vi "save_bin2.vi"(4 "error in":errorcluster, 5 "xz":T1, 7 "start path":path) -> (0 "error out":errorcluster, 1 "timestamp":timestamp, 3 "file path out":path)   [LabVIEW 2010]
uses:
  lib/Global 2.vi
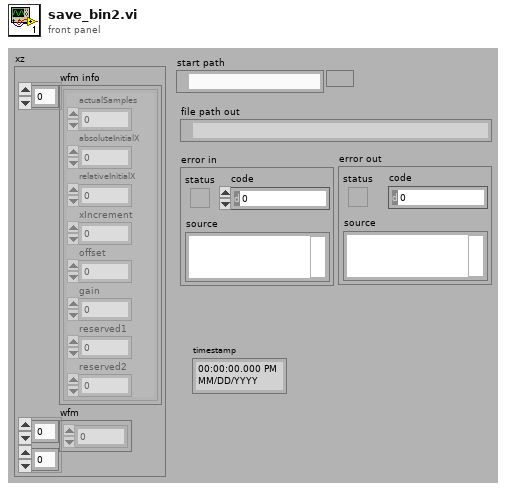
[diagram p1: front panel]
types:
  T1 = cluster{"wfm info":cluster{"actualSamples":i32, "absoluteInitialX":dbl, "relativeInitialX":dbl, "xIncrement":dbl, "offset":dbl, "gain":dbl, "reserved1":dbl, "reserved2":dbl}[], "wfm":i16[][]}
  T2 = enum16{"open", "open or create", "create or replace", "create", "open (read-only)"}
  T3 = cluster{"actualSamples":i32, "absoluteInitialX":dbl, "relativeInitialX":dbl, "xIncrement":dbl, "offset":dbl, "gain":dbl, "reserved1":dbl, "reserved2":dbl}[]
  T4 = cluster{"actualSamples":i32, "absoluteInitialX":dbl, "relativeInitialX":dbl, "xIncrement":dbl, "offset":dbl, "gain":dbl, "reserved1":dbl, "reserved2":dbl}
  T5 = cluster{"name":enum16{"sync", "phase_a", "phase_b", "phase_c", "ground"}, "num":i32, "Numeric":i32}[]
  T6 = enum16{"sync", "phase_a", "phase_b", "phase_c", "ground"}
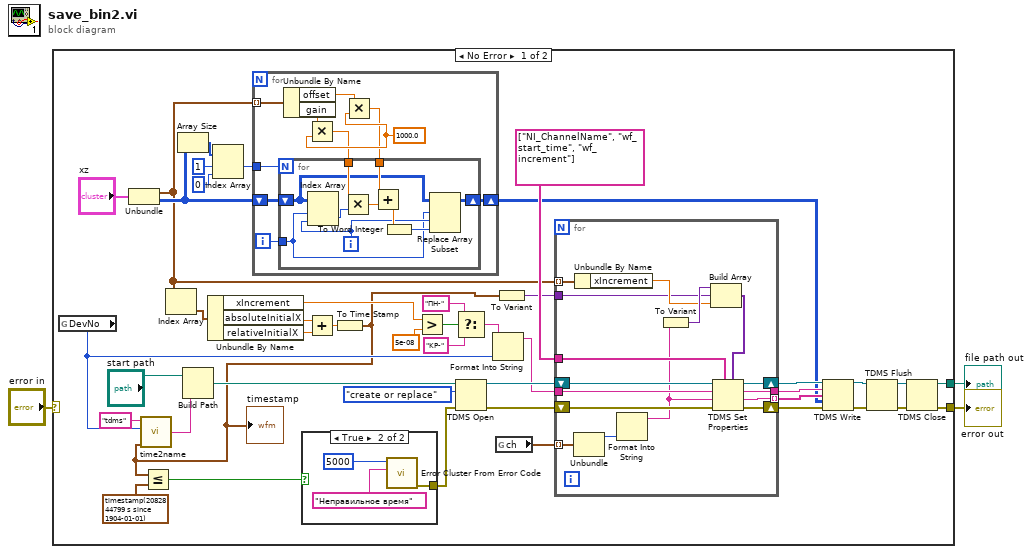
[diagram p0: block diagram]
diagram:
  n1 = case shown="No Error" "error in" {
    selector: "error in" -> [_ w87]
    tunnel: [w45 w87] -> w3
    tunnel: [w44 _] -> w2
    frame No Error {
      n2 = global read "Global 2.vi" "DevNo"() -> (w22:i32)
      n3 = Unbundle("xz") -> ("wfm info"=w26:T3, "wfm"=w47:i16[][])
      n4 = Index Array(array=w26) -> (element=w25:T4)  [unwired: 1 in]
      n5 = Array Size(array=w47) -> (size(s)=w39:i32[])
      n6 = Unbundle By Name(w25) -> ("xIncrement"=w24:dbl, "absoluteInitialX"=w8:dbl, "relativeInitialX"=w9:dbl)
      n7 = Index Array(array=w39, index #1=1 ("index"), index #2=0 ("index")) -> (element #1=w41:i32)  [unwired: 1 out]
      n8 = for {
        tunnel: w26 -> [w74] mode=indexing
        shift-right: [w70] -> w11
        shift-left: w47 -> [w72]
        tunnel: w41 -> [w69]
        i -> [w71]
        w73 = 1000.0
        n9 = Unbundle By Name(w74) -> ("offset"=w75:dbl, "gain"=w76:dbl)
        n10 = Multiply(x=w76, y=w73) -> (x*y=w67:dbl)
        n11 = Multiply(x=w75, y=w73) -> (x*y=w68:dbl)
        n12 = for {
          N: w69 -> [_]
          tunnel: w67 -> [w84]
          tunnel: w68 -> [w83]
          tunnel: w71 -> [w77]
          shift-right: [w79] -> w70
          shift-left: w72 -> [w81]
          i -> [w78]
          n13 = Index Array(array=w81, index (row)=w77, index (col)=w78) -> (element=w82:i16)
          n14 = Multiply(x=w84, y=w82) -> (x*y=w86:dbl)
          n15 = Add(x=w83, y=w86) -> (x+y=w85:dbl)
          n16 = To Word Integer(number=w85) -> (16bit integer=w80:i16)
          n17 = Replace Array Subset(array=w81, new element=w80, index (row)=w77, index (col)=w78) -> (w79:i16[][])
        }
      }
      n18 = Add(x=w8, y=w9) -> (x+y=w7:dbl)
      n19 = To Time Stamp(1:w7) -> (0:w5:timestamp)
      "timestamp" <- w5
      n20 = call "time2name.vi"("timestamp"=w5, "DevNo"=w22, "ext"="tdms") -> ("String"=w35:string)  [unwired: 1 in]
      n21 = Less Or Equal?(x=w5, y=timestamp(2082844799 s since 1904-01-01) ("timestamp")) -> (x <= y?=w31:bool)
      n22 = Build Path(base path="start path", name or relative path=w35) -> (appended path=w33:path)
      n23 = case shown="True" w31 {
        tunnel: [_ w48] -> w23
        frame False {
        }
        frame True {
          n24 = call <vilib>:"Error Cluster From Error Code.vi"("error message (\"\")"="Неправильное время" ("string"), "error code (0)"=5000) -> ("error out"=w48:errorcluster)  [unwired: 7 in]
        }
      }
      n25 = Greater?(x=w24, y=5e-08 ("dt")) -> (0:w28:bool)
      n26 = Select(t="ПН-" ("ext"), s=w28, f="KP-" ("ext")) -> (s? t:f=w6:string)
      n27 = TDMS Open(8:w23, 10:T2."create or replace" ("operation (0:open)"), 11:w33) -> (0:w20:errorcluster, 3:w19:refnum<k34>)  [unwired: 3 in]
      n28 = Format Into String(initial string=w6, w22) -> (resulting string=w18:string)  [unwired: 2 in, 1 out]
      n29 = global read "Global 2.vi" "ch"() -> (w10:T5)
      n30 = To Variant(anything=w5) -> (Variant=w4:variant)
      n31 = for {
        shift-right: [w66] -> w17
        shift-left: w20 -> [w65]
        shift-right: [w64] -> w16
        shift-left: w19 -> [w63]
        tunnel: w26 -> [w62] mode=indexing
        tunnel: string[] ["NI_ChannelName", "wf_start_time", "wf_increment"] -> [w60]
        tunnel: w18 -> [w59]
        tunnel: [w56] -> w14
        tunnel: [w55] -> w15 mode=indexing
        tunnel: w10 -> [w53] mode=indexing
        tunnel: w4 -> [w51]
        n32 = Unbundle(w53) -> ("name"=w54:T6)  [unwired: 2 out]
        n33 = Unbundle By Name(w62) -> ("xIncrement"=w57:dbl)
        n34 = Format Into String(w54) -> (resulting string=w52:string)  [unwired: 3 in, 1 out]
        n35 = To Variant(anything=w52) -> (Variant=w58:variant)
        n36 = Build Array(w58, w51, w57) -> (w61:variant[])
        n37 = TDMS Set Properties(5:w61, 7:w60, 8:w65, 9:w52, 10:w59, 11:w63) -> (0:w66:errorcluster, 1:w55:string, 2:w56:string, 3:w64:refnum<k34>)
      }
      n38 = TDMS Write(0:w16, 5:w14, 7:w15, 9:w11, 11:w17) -> (4:w12:refnum<k34>, 15:w13:errorcluster)  [unwired: 1 in, 2 out]
      n39 = TDMS Flush(4:w13, 7:w12) -> (0:w37:errorcluster, 3:w38:refnum<k34>)
      n40 = TDMS Close(8:w37, 11:w38) -> (0:w45:errorcluster, 3:w44:path)
    }
    frame Error {
    }
  }
  "error out" <- w3
  "file path out" <- w2
